vi "Rotate.vi"(8 "error in (no error)":errorcluster, 10 "Angle (deg)":dbl, 11 "IRotatable in":refnum<class "IRotatable.lvclass">) -> (0 "error out":errorcluster, 3 "IRotatable out":refnum<class "IRotatable.lvclass">)   [LabVIEW 2021, in "Picture2D.lvlib" / "IRotatable.lvclass"]
uses:
  IRotatable.lvclass
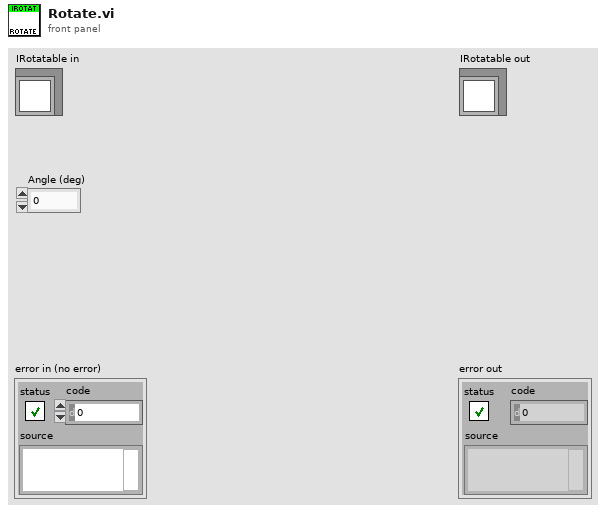
[diagram p1: front panel]
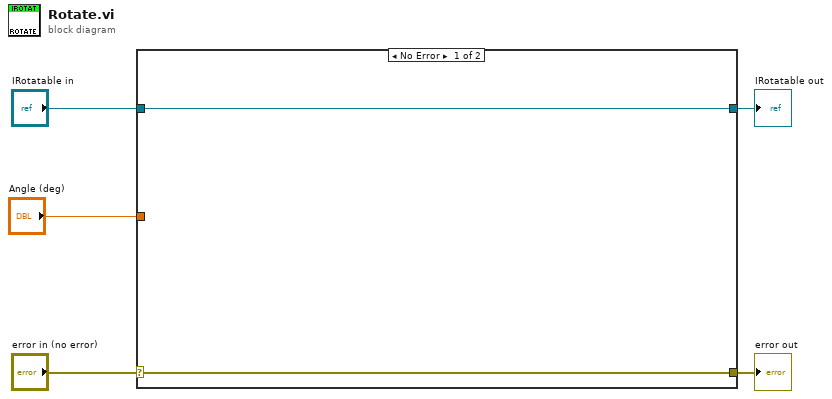
[diagram p0: block diagram]
diagram:
  n1 = case shown="No Error" "error in (no error)" {
    selector: "error in (no error)" -> [w6 w9]
    tunnel: [w6 w9] -> w4
    tunnel: [w7 w8] -> w2
    tunnel: "IRotatable in" -> [w7 w8]
    tunnel: "Angle (deg)" -> [_ _]
    frame No Error {
    }
    frame Error {
    }
  }
  "error out" <- w4
  "IRotatable out" <- w2
